vi "CloseCOM.vi"(11 "PN532 COM Port":refnum<visa-resource-name>) -> (0 "Error Out":errorcluster)   [LabVIEW 2012, in "NFC Driver.lvlib"]
doc: "This VI closes the communication session with the PN532."
uses:
  NFC Driver.lvlib
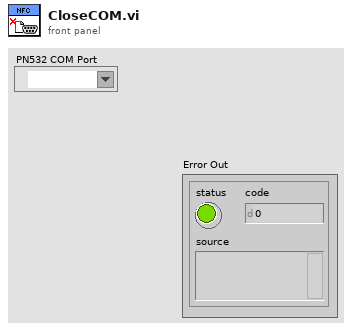
[diagram p1: front panel]
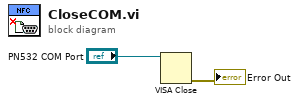
[diagram p0: block diagram]
diagram:
  n1 = VISA Close(VISA resource name="PN532 COM Port") -> (error out=→"Error Out":errorcluster)  [unwired: 1 in]
